vi "Boxplot - Compute Boxplot data.vi"(5 "Box Space":dbl=5.0, 7 "Box Width":dbl=10.0, 10 "Plot number":dbl format="%#.6f", 11 "Raw data":dbl[](array[numeric]) format="%#.6f") -> (2 "Boxplot":cluster{dbl[], dbl[]}[](graph))   [LabVIEW 2023]
doc: "Computes the data for the boxplot."
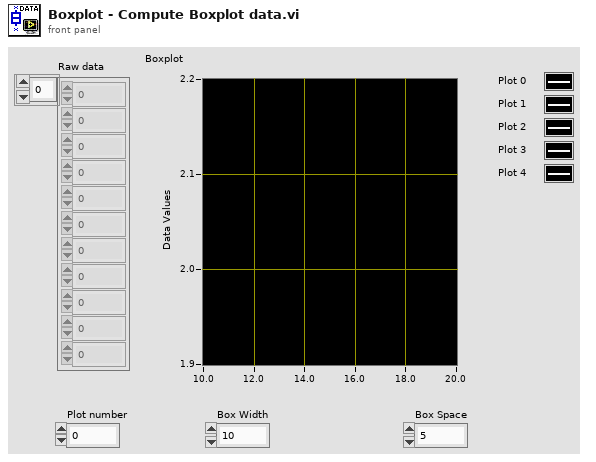
[diagram p1: front panel]
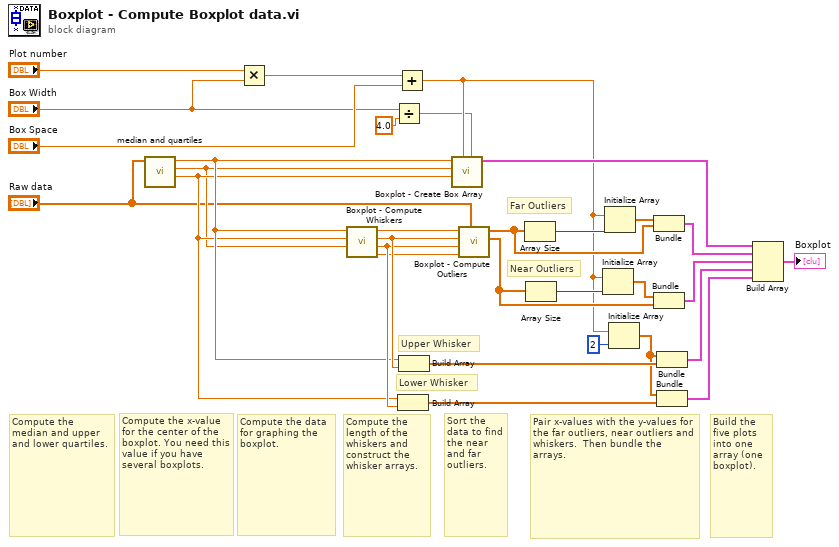
[diagram p0: block diagram]
diagram:
  # "Sort the data to find the near and far outliers."
  # "Compute the length of the whiskers and construct the whisker arrays."
  # "Compute the data for graphing the boxplot."
  # "Compute the x-value for the center of the boxplot. You need this value if you have several boxplots."
  # "Compute the median and upper and lower quartiles."
  # "Build the  five plots into one array (one boxplot)."
  # "Near Outliers"
  # "Far Outliers"
  # "Pair x-values with the y-values for the far outliers, near outliers and whiskers.  Then bundle the arrays."
  # "Lower Whisker"
  # "Upper Whisker"
  n1 = call "median and quartiles.vi"("Data"="Raw data") -> ("Lower quartile (LQ)"=w10:dbl, "Median"=w8:dbl, "Upper quartile (UQ)"=w11:dbl)  [unwired: 8 in]
  n2 = Multiply(x="Plot number", y="Box Width") -> (x*y=w7:dbl)
  n3 = call "Boxplot - Compute Whiskers.vi"("Median"=w8, "Lower quartile (LQ)"=w10, "Upper quartile (UQ)"=w11) -> ("L2"=w17:dbl, "L1"=w18:dbl, "U1"=w20:dbl, "U2"=w19:dbl)  [unwired: 5 in]
  n4 = Divide(x="Box Width", y=4.0) -> (x/y=w3:dbl)
  n5 = Add(x=w7, y="Box Space") -> (x+y=w5:dbl)
  n6 = Build Array(w10, w18) -> (w23:dbl[])
  n7 = Build Array(w11, w20) -> (w24:dbl[])
  n8 = call "Boxplot - Create Box Array.vi"("delta x"=w3, "x"=w5, "Lower quartile (LQ)"=w10, "Median"=w8, "Upper quartile (UQ)"=w11) -> ("XY Graph"=w16:cluster{dbl[], dbl[]})  [unwired: 6 in]
  n9 = call "Boxplot - Compute Outliers.vi"("Raw data"="Raw data", "L2"=w17, "L1"=w18, "U1"=w20, "U2"=w19) -> ("Near outliers"=w27:dbl[], "Far outliers"=w26:dbl[])  [unwired: 5 in]
  n10 = Array Size(array=w26) -> (size(s)=w31:i32)
  n11 = Array Size(array=w27) -> (size(s)=w30:i32)
  n12 = Initialize Array(w5, w30) -> (w28:dbl[])
  n13 = Initialize Array(w5, w31) -> (w29:dbl[])
  n14 = Initialize Array(w5, 2 ("dimension size")) -> (w22:dbl[])
  n15 = Bundle(w29, "Far outliers"=w26) -> (w15:cluster{dbl[], "Far outliers":dbl[]})  [unwired: 1 in]
  n16 = Bundle(w28, "Near outliers"=w27) -> (w14:cluster{dbl[], "Near outliers":dbl[]})  [unwired: 1 in]
  n17 = Bundle(w22, w24) -> (w13:cluster{dbl[], dbl[]})  [unwired: 1 in]
  n18 = Bundle(w22, w23) -> (w12:cluster{dbl[], dbl[]})  [unwired: 1 in]
  n19 = Build Array(w16, w15, w14, w13, w12) -> (→"Boxplot":cluster{dbl[], "Near outliers":dbl[]}[])
